vi "ArmPathPlanPreview.vi"(0 "AvoidancePolygon":T1) -> (1 "Rotation Path":T4[](array[typedef]) {"Time (ms)" items=["TrajectoryDuration_0ms"=0, "TrajectoryDuration_5ms"=5, "TrajectoryDuration_10ms"=10, "TrajectoryDuration_20ms"=20, "TrajectoryDuration_30ms"=30, "TrajectoryDuration_40ms"=40, "TrajectoryDuration_50ms"=50, "TrajectoryDuration_100ms"=100]}, 2 "Extension Path":T4[](array[typedef]) {"Time (ms)" items=["TrajectoryDuration_0ms"=0, "TrajectoryDuration_5ms"=5, "TrajectoryDuration_10ms"=10, "TrajectoryDuration_20ms"=20, "TrajectoryDuration_30ms"=30, "TrajectoryDuration_40ms"=40, "TrajectoryDuration_50ms"=50, "TrajectoryDuration_100ms"=100]}, 3 "Go":bool)   [LabVIEW 2017]
uses:
  General/PathPlanning/TypeDefs/Point2D.ctl
  General/MotionProfiling/TypeDefs/MotionProfileGeneratorParams.ctl
  <vilib>/Rock Robotics/WPI/ThirdParty/Phoenix-LabVIEW/Motor Controller/Controls/CTRE_Phoenix_MotorControl_TrajectoryPointTimeDur.ctl
  General/MotionProfiling/TypeDefs/TrajectoryPoint.ctl
  General/PathPlanning/TypeDefs/Polygon2D.ctl
  ArgosLib/Signal Processing/TypeDefs/EdgeDetector_Type.ctl
  ArgosLib/ArgosLib.lvlib
panel:
  out "Rotation Path Graph":T3(graph)
  in  "Preview?":bool
  in  "Send Path Plan":bool
  out "Extension Path Graph":T3(graph)
  in  "Reverse Direction":bool
  in  "MotionProfileGeneratorParameters":T6={"Trajectory Point Interval (ms)"=10, "Maximum Travel Speed (units/s)"=0.0, "Velocity Ramp Time (ms)"=0.0, "Acceleration Ramp Time (ms)"=1.0} {"Acceleration Ramp Time (ms)" min=1.0; "Velocity Ramp Time (ms)" min=1.0; "Maximum Travel Speed (units/s)" min=0.0; "Trajectory Point Interval (ms)" items=["TrajectoryDuration_0ms"=0, "TrajectoryDuration_5ms"=5, "TrajectoryDuration_10ms"=10, "TrajectoryDuration_20ms"=20, "TrajectoryDuration_30ms"=30, "TrajectoryDuration_40ms"=40, "TrajectoryDuration_50ms"=50, "TrajectoryDuration_100ms"=100]}
  in  "EndPoint":T2
  in  "StartPoint":T2
  in  "PathPointSpacing (in)":dbl=0.25
  in  "MaxArmLength":dbl=68.0
  in  "MinArmLength":dbl=44.0
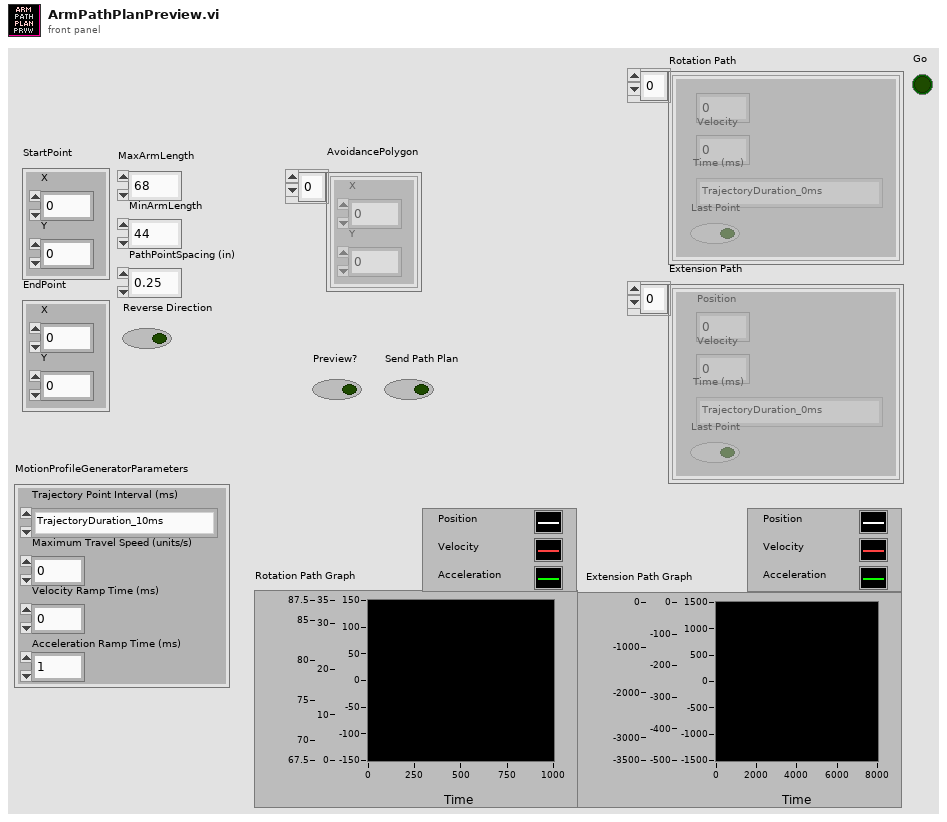
[diagram p1: front panel]
types:
  T1 = typedef "Polygon2D.ctl" = T2[]
  T2 = typedef "Point2D.ctl" = cluster{"X":dbl, "Y":dbl}
  T3 = cluster{dbl, "Trajectory Point Interval (ms)":i32, dbl[][]}
  T4 = typedef "TrajectoryPoint.ctl" = cluster{"Position ":dbl, "Velocity ":dbl, "Time (ms)":T5, "Last Point":bool}
  T5 = typedef "CTRE_Phoenix_MotorControl_TrajectoryPointTimeDur.ctl" = i32
  T6 = typedef "MotionProfileGeneratorParams.ctl" = cluster{"Trajectory Point Interval (ms)":T5, "Maximum Travel Speed (units/s)":dbl, "Velocity Ramp Time (ms)":dbl, "Acceleration Ramp Time (ms)":dbl}
  T7 = typedef "ArgosLib.lvlib/EdgeDetector_Type.ctl" = enum16{"RisingEdge", "FallingEdge", "Both"}
  T8 = cluster{dbl, "Trajectory Point Interval (ms)":T5, dbl[][]}
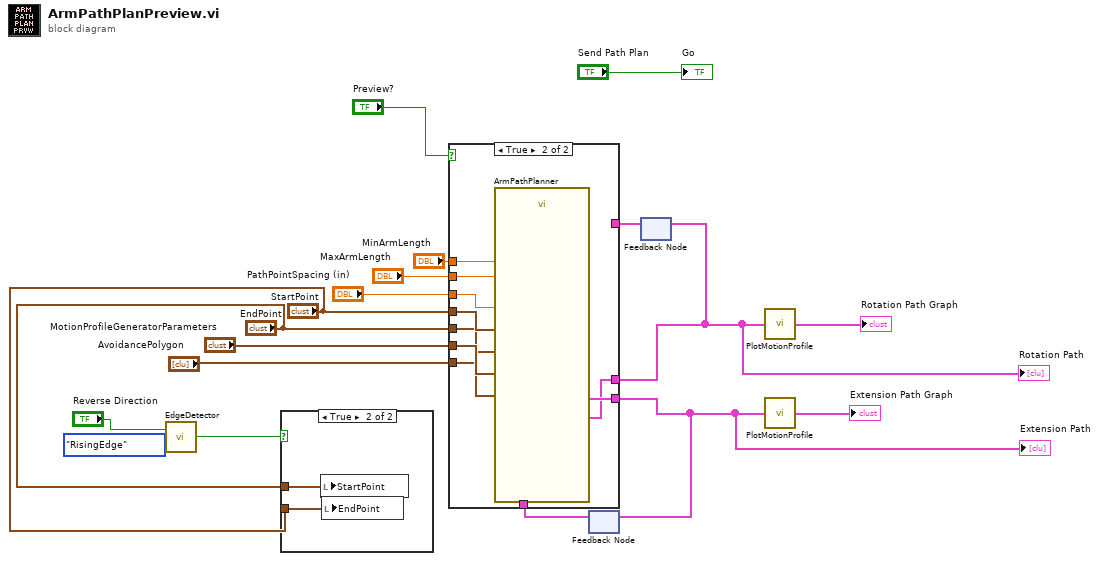
[diagram p0: block diagram]
diagram:
  n1 = call "EdgeDetector.vi"("DetectorType"=EdgeDetector_Type."RisingEdge", "Input"="Reverse Direction") -> ("Edge"=w14:bool)
  n2 = case shown="True" w14 {
    tunnel: "StartPoint" -> [_ w20]
    tunnel: "EndPoint" -> [_ w19]
    frame False {
    }
    frame True {
      n3 = local write "StartPoint"(w19) -> ()
      n4 = local write "EndPoint"(w20) -> ()
    }
  }
  n5 = feedback #1() -> (w5:T4[])  [unwired: 1 in]
  n6 = feedback #2() -> (w3:T4[])  [unwired: 1 in]
  n7 = case shown="True" "Preview?" {
    tunnel: "MinArmLength" -> [_ w31]
    tunnel: "MaxArmLength" -> [_ w30]
    tunnel: "PathPointSpacing (in)" -> [_ w29]
    tunnel: "MotionProfileGeneratorParameters" -> [_ w28]
    tunnel: "StartPoint" -> [_ w27]
    tunnel: "EndPoint" -> [_ w26]
    tunnel: [w21 w24] -> w4
    tunnel: [w22 w25] -> w6
    tunnel: w5 -> [w22 _]
    tunnel: w3 -> [w21 _]
    tunnel: "AvoidancePolygon" -> [_ w23]
    frame False {
    }
    frame True {
      n8 = call "ArmPathPlanner.vi"("StartPoint"=w27, "EndPoint"=w26, "PathPointSpacing (in)"=w29, "MinArmLength"=w31, "MaxArmLength"=w30, "AvoidancePolygon"=w23, "MotionProfileGeneratorParameters"=w28) -> ("RotatePath"=w24:T4[], "ExtendPath"=w25:T4[])  [unwired: 9 in, 2 out]
    }
  }
  "Rotation Path" <- w4
  "Extension Path" <- w6
  n9 = feedback-in #1(w6) -> ()
  n10 = feedback-in #2(w4) -> ()
  n11 = call "PlotMotionProfile.vi"("Trajectory Points"=w4) -> ("MotionProfileGraph"=→"Rotation Path Graph":T8)
  n12 = call "PlotMotionProfile.vi"("Trajectory Points"=w6) -> ("MotionProfileGraph"=→"Extension Path Graph":T8)
  "Go" <- "Send Path Plan"
